vi "Triggering.vi"   [LabVIEW 2009, in "MicroDAQ.lvlib"]
uses:
  <instrlib>/MicroDAQ/MicroDAQ.lvlib
  <instrlib>/MicroDAQ/Channel/Analog Input/Analog Input.lvclass
  <instrlib>/MicroDAQ/Channel/Analog Output/Analog output.lvclass
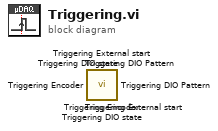
[diagram p0: block diagram]
diagram:
  n1 = call <instrlib>:"Triggering Encoder.vi"() -> ()  [unwired: 10 in, 2 out]
  n2 = call <instrlib>:"Triggering DIO Pattern.vi"() -> ()  [unwired: 10 in, 2 out]
  n3 = call <instrlib>:"Triggering Encoder.vi"() -> ()  [unwired: 10 in, 2 out]
  n4 = call <instrlib>:"Triggering DIO Pattern.vi"() -> ()  [unwired: 10 in, 2 out]
  n5 = call <instrlib>:"Triggering DIO state.vi"() -> ()  [unwired: 10 in, 2 out]
  n6 = call <instrlib>:"Triggering External start.vi"() -> ()  [unwired: 10 in, 2 out]
  n7 = call <instrlib>:"Triggering DIO state.vi"() -> ()  [unwired: 10 in, 2 out]
  n8 = call <instrlib>:"Triggering External start.vi"() -> ()  [unwired: 10 in, 2 out]
